vi "Thermal Chamber Controller_DQMH teardown.vi"(8 "error in (no error)":errorcluster) -> (0 "error out":errorcluster)   [LabVIEW 2015]
doc: "_____\nCreated using Delacor QMH Event Scripter 4.0.0.68."
uses:
  Libraries/Thermal Chamber Controller_DQMH/Thermal Chamber Controller_DQMH.lvlib
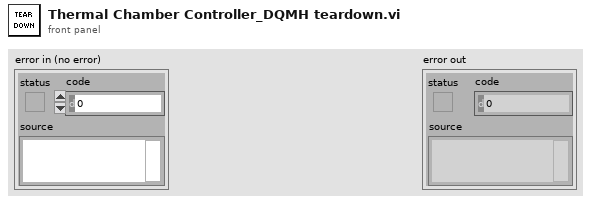
[diagram p1: front panel]
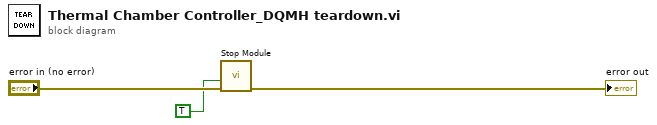
[diagram p0: block diagram]
diagram:
  n1 = call "Stop Module.vi"("error in (no error)"="error in (no error)", "Wait for Module to Stop? (F)"=TRUE) -> ("error out"=→"error out":errorcluster)  [unwired: 9 in]
